vi "Initialize.vi"(8 "error in (no error)":errorcluster, 9 "Reset (True)":bool=TRUE, 10 "ID Query (True)":bool=TRUE, 11 "VISA resource name in":refnum<visa-resource-name>) -> (0 "error out":errorcluster, 3 "VISA resource name out":refnum<visa-resource-name>)   [LabVIEW 2022 SP3, in "usbtmc_scpi_labtool.lvlib"]
uses:
  usbtmc_scpi_labtool.lvlib
panel:
  in  "delay before read (ms)":u32=500
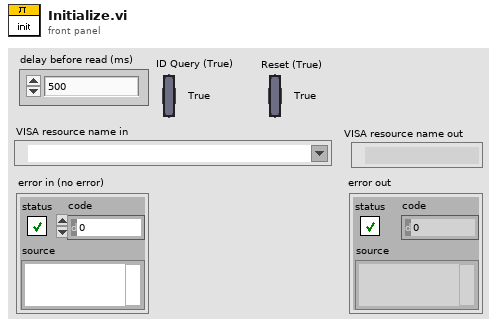
[diagram p1: front panel]
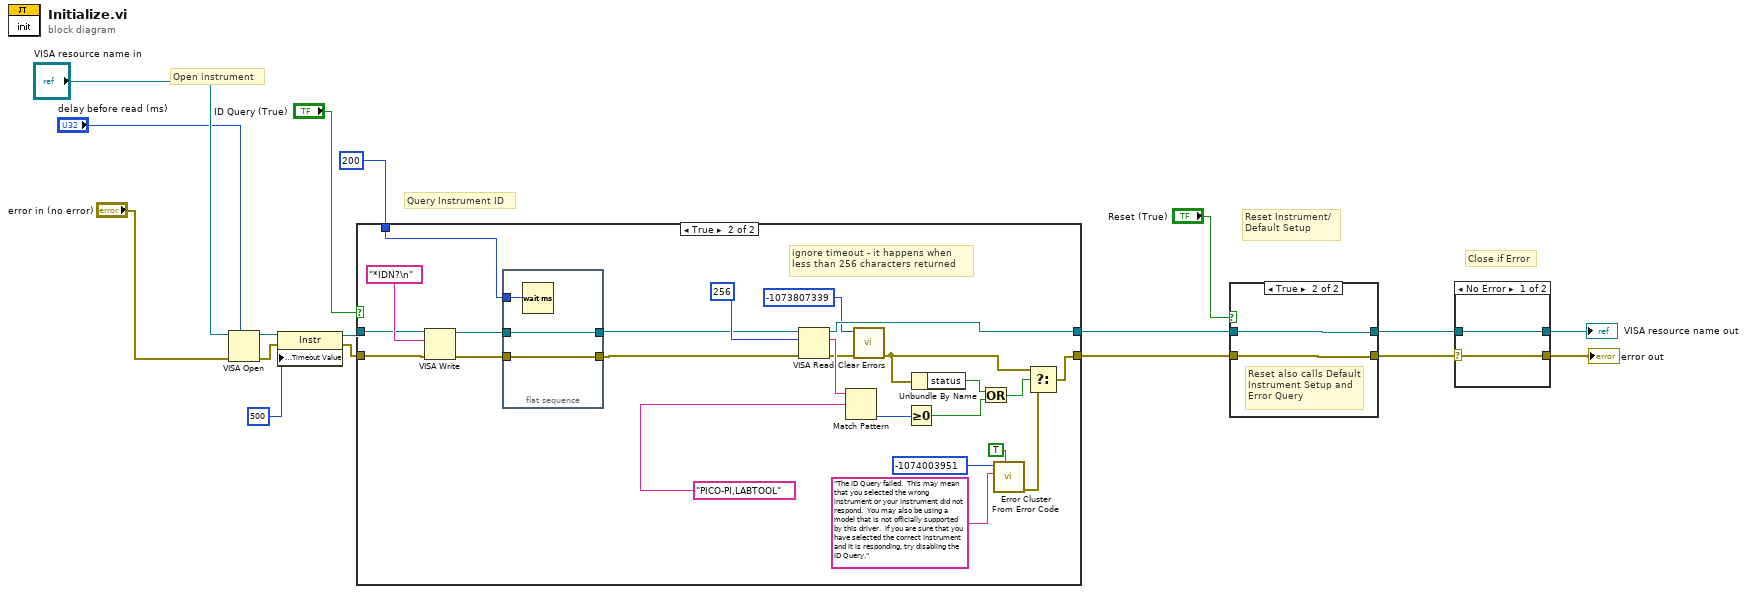
[diagram p0: block diagram]
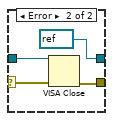
[diagram p4: hidden frame]
diagram:
  # "Query Instrument ID"
  # "Reset Instrument/\nDefault Setup"
  # "Open instrument"
  # "Close if Error"
  n1 = VISA Open(timeout (0)="delay before read (ms)", error in (no error)="error in (no error)", VISA resource name="VISA resource name in") -> (VISA resource name=w4:refnum<visa-resource-name>, error out=w3:errorcluster)  [unwired: 2 in]
  n2 = property class="Instr"(reference=w4, error in=w3, "General Settings:Timeout Value"=u32 500) -> (reference out=w1:refnum<visa-resource-name>, error out=w2:errorcluster)
  n3 = case shown="True" "ID Query (True)" {
    tunnel: [w18 w43] -> w14
    tunnel: [w19 w42] -> w15
    tunnel: w1 -> [w19 w26]
    tunnel: w2 -> [w18 w31]
    tunnel: 200 -> [_ w30]
    frame False {
    }
    frame True {
      # "ignore timeout - it happens when \nless than 256 characters returned"
      n4 = VISA Write(VISA resource name=w26, write buffer="*IDN?\n" ("Command"), error in (no error)=w31) -> (VISA resource name out=w29:refnum<visa-resource-name>, error out=w28:errorcluster)  [unwired: 1 out]
      n5 = flat-sequence {
        tunnel: w30 -> [w46]
        tunnel: w29 -> [w45]
        tunnel: w28 -> [w44]
        tunnel: [w45] -> w21
        tunnel: [w44] -> w20
        frame #0 {
          n6 = Wait (ms)(milliseconds to wait=w46) -> ()  [unwired: 1 out]
        }
      }
      n7 = VISA Read(VISA resource name=w21, byte count=256, error in (no error)=w20) -> (VISA resource name out=w42:refnum<visa-resource-name>, read buffer=w41:string, error out=w24:errorcluster)  [unwired: 1 out]
      n8 = Match Pattern(string=w41, regular expression="PICO-PI,LABTOOL") -> (offset past match=w35:i32)  [unwired: 4 out]
      n9 = call <vilib>:"Clear Errors.vi"("error in (no error)"=w24, "specific error code to clear (0: all)"=-1073807339) -> ("error out"=w23:errorcluster)  [unwired: 4 in, 1 out]
      n10 = Greater Or Equal To 0?(x=w35) -> (x >= 0?=w33:bool)
      n11 = Unbundle By Name(w23) -> ("status"=w34:bool)
      n12 = Or(x=w34, y=w33) -> (x .or. y?=w32:bool)
      n13 = call <vilib>:"Error Cluster From Error Code.vi"("show call chain? (False)"=TRUE, "error message (\"\")"="The ID Query failed.  This may mean that you selected the wrong instrument or your instrument did not respond.  You may also be using a model that is not officially supported by this driver.  If you are sure that you have selected the correct instrument and it is responding, try disabling the ID Query." ("Source (VI Name)"), "error code (0)"=-1074003951 ("Code")) -> ("error out"=w39:errorcluster)  [unwired: 1 in, 5 out]
      n14 = Select(t=w23, s=w32, f=w39) -> (s? t:f=w43:errorcluster)
    }
  }
  n15 = case shown="True" "Reset (True)" {
    tunnel: w14 -> [w47 w49]
    tunnel: [w47 w49] -> w10
    tunnel: w15 -> [w48 w50]
    tunnel: [w48 w50] -> w11
    frame False {
    }
    frame True {
      # "Reset also calls Default Instrument Setup and Error Query"
    }
  }
  n16 = case shown="No Error" w10 {
    selector: w10 -> [w51 w55]
    tunnel: w11 -> [w52 w54]
    tunnel: [w52 refnum<visa-resource-name> refnum ("VISA resource name out")] -> w17
    tunnel: [w51 w53] -> w16
    frame No Error {
    }
    frame Error {
      n17 = VISA Close(VISA resource name=w54, error in (no error)=w55) -> (error out=w53:errorcluster)
    }
  }
  "error out" <- w16
  "VISA resource name out" <- w17
